vi "RT - FPGA Loop Test.vi"() -> ()   [LabVIEW 2018]
panel:
  out "Array 2":dbl[](array[numeric])
  out "size(s) 2":i32
  out "Array":bool[](array[boolean])
  out "size(s)":i32
  out "loop no":i32
  out "appended array":bool[](array[boolean])
  out "subarray":bool[](array[boolean])
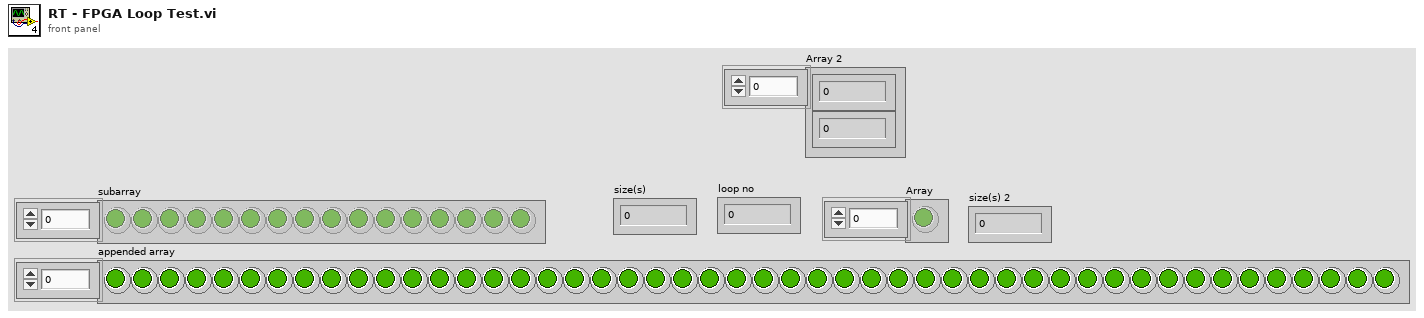
[diagram p1: front panel]
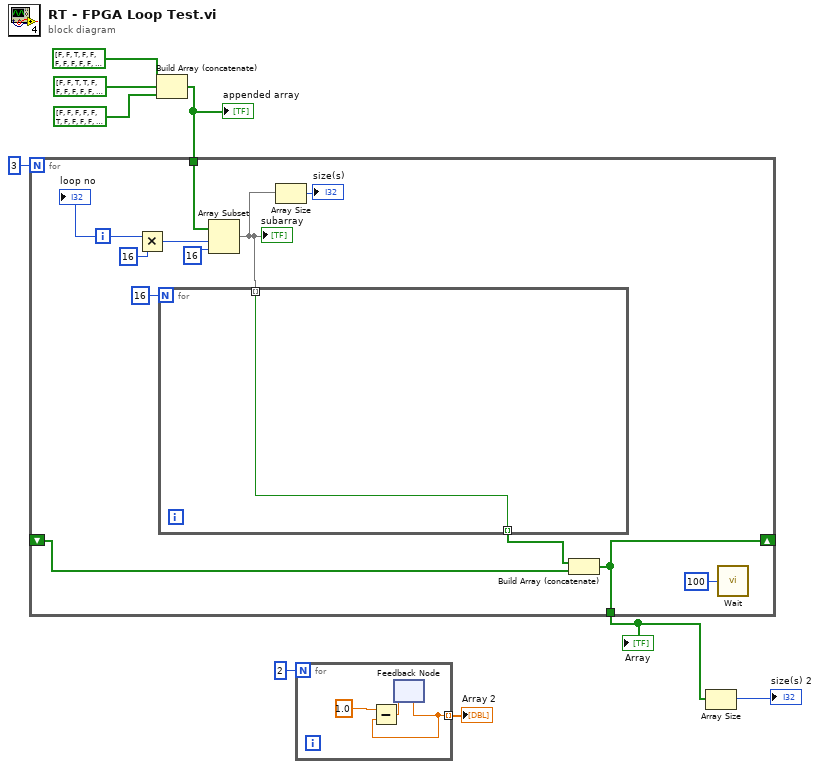
[diagram p0: block diagram]
diagram:
  n1 = Build Array (concatenate)(bool[] [FALSE, FALSE, TRUE, FALSE, FALSE, FALSE, FALSE, FALSE, FALSE, FALSE, FALSE, FALSE, FALSE, FALSE, FALSE, FALSE] ("ADC 3 W"), bool[] [FALSE, FALSE, TRUE, TRUE, FALSE, FALSE, FALSE, FALSE, FALSE, FALSE, FALSE, FALSE, FALSE, FALSE, FALSE, FALSE] ("ADC 4 W"), bool[] [FALSE, FALSE, FALSE, FALSE, FALSE, TRUE, FALSE, FALSE, FALSE, FALSE, FALSE, FALSE, FALSE, FALSE, FALSE, FALSE] ("ADC 1 W")) -> (w6:bool[])
  "appended array" <- w6
  n2 = for {
    N: 3 -> [_]
    tunnel: w6 -> [w18]
    tunnel: [w11] -> w4
    shift-right: [w11] -> _
    shift-left: _ -> [w10]
    i -> [w17]
    n3 = Multiply(x=w17, y=16) -> (x*y=w21:i32)
    n4 = Array Subset(array=w18, index=w21, length=16) -> (w13:bool[])
    "subarray" <- w13
    n5 = for {
      N: 16 -> [_]
      tunnel: w13 -> [w22] mode=indexing
      tunnel: [w22] -> w12 mode=indexing
    }
    n6 = Array Size(array=w13) -> (size(s)=→"size(s)":i32)
    n7 = Build Array (concatenate)(w12, w10) -> (w11:bool[])
    n8 = call "Wait"("Count(mSec)"=u32 100) -> ()  [unwired: 1 out]
    "loop no" <- w17
  }
  "Array" <- w4
  n9 = for {
    N: 2 -> [_]
    tunnel: [w23] -> w1 mode=indexing
    n10 = feedback #1() -> (w23:dbl)  [unwired: 1 in]
    n11 = Subtract(x=1.0, y=w23) -> (x-y=w24:dbl)
    n12 = feedback-in #1(w24) -> ()
  }
  "Array 2" <- w1
  n13 = Array Size(array=w4) -> (size(s)=→"size(s) 2":i32)
